vi "NI GetWaveform Queue.vi"(0 "Acq ID In":refnum<k15>, 1 "File Array":refnum<file>[](array[refnum]), 2 "timeout":dbl=1.0, 5 "Num Samps":i32=1000, 7 "Channel array":string[](array[string])=["0", "1"], 9 "Num Segs":i32=1, 11 "error in":errorcluster, 12 "Reverse?":bool, 13 "File Array":string[](array[string])) -> (4 "Acq ID Out":refnum<k15>, 15 "error out":errorcluster)   [LabVIEW 2022 SP3]
uses:
  <instrlib>/niScope/Acquire/Fetch/niScope Multi Fetch Binary 8.vi
  -ScanSystem/DataHandling/ReverseDataI8.vi
panel:
  # "Mujst convert data at output for Integers"
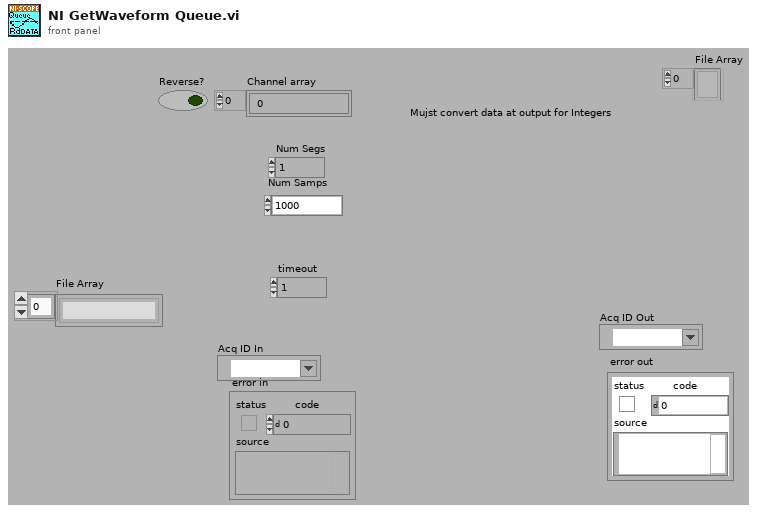
[diagram p1: front panel]
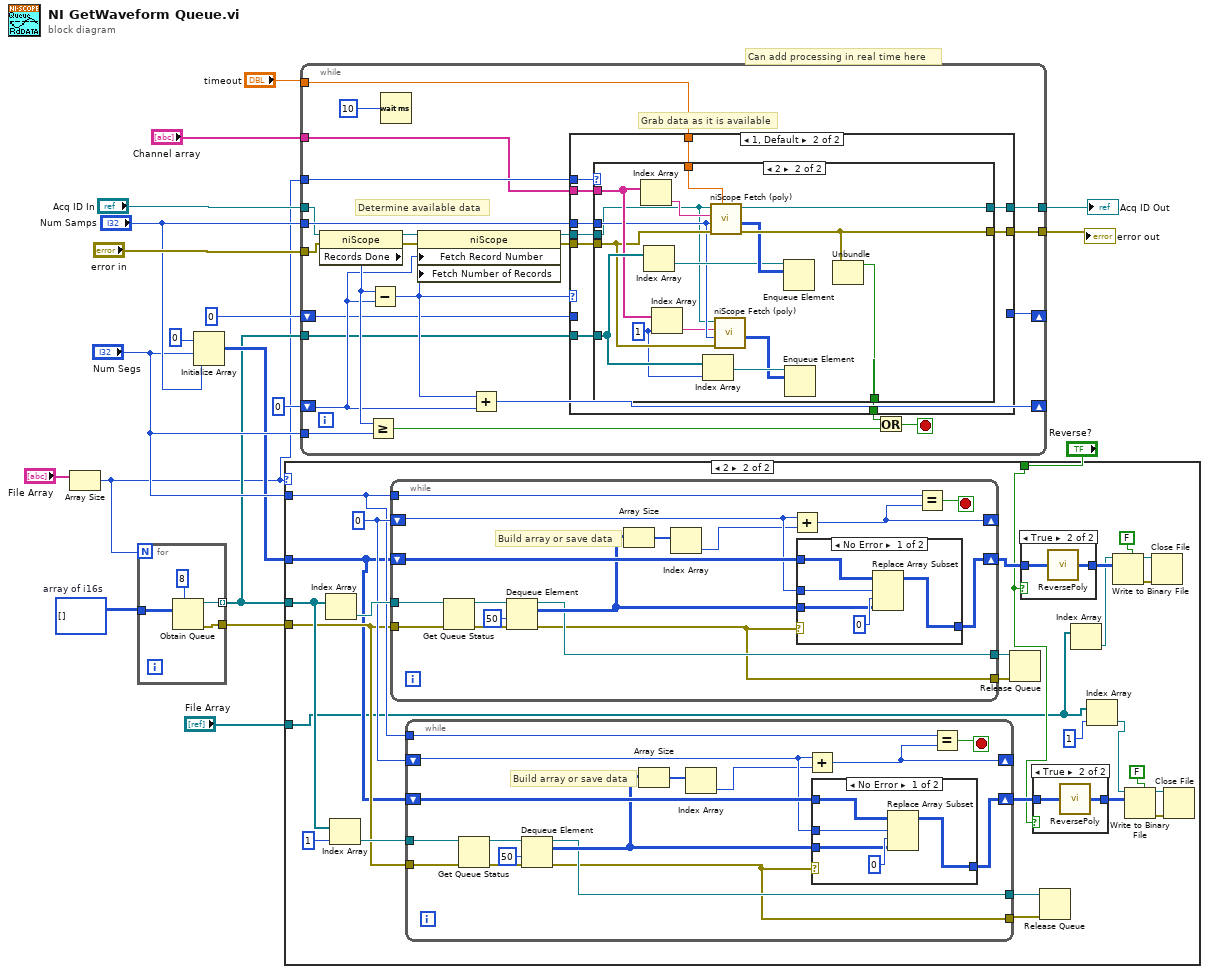
[diagram p0: block diagram]
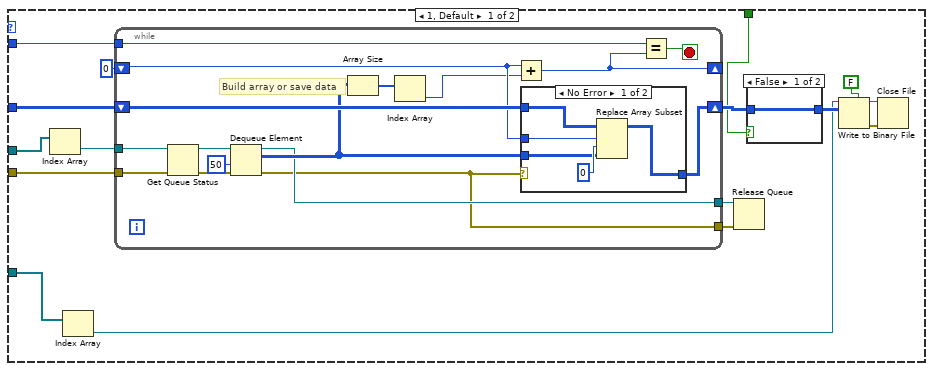
[diagram p2: hidden frame]
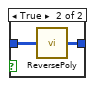
[diagram p3: hidden frame]
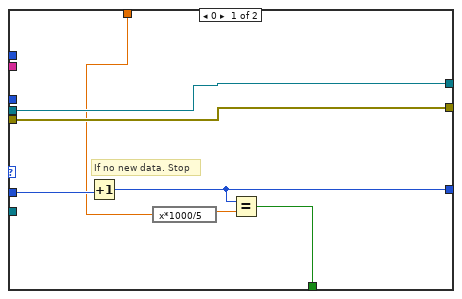
[diagram p9: hidden frame]
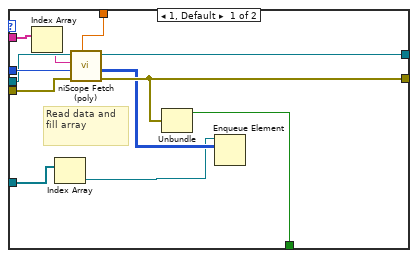
[diagram p10: hidden frame]
diagram:
  w11 = i8[][] []  # array of i16s
  # "Can add processing in real time here"
  n1 = Array Size(array="File Array") -> (size(s)=w1:i32)
  n2 = for {
    N: w1 -> [_]
    tunnel: w11 -> [w23]
    tunnel: [w21] -> w10
    tunnel: [w20] -> w8 mode=indexing
    n3 = Obtain Queue(max queue size (-1, unlimited)=8, element data type=w23) -> (queue out=w20:refnum<queue>, error out=w21:errorcluster)  [unwired: 2 in, 2 out]
  }
  n4 = Initialize Array(i8 0, "Num Segs", "Num Samps") -> (w9:i8[][])
  n5 = case shown="2" w1 {
    tunnel: "Num Segs" -> [w39 w82]
    tunnel: w10 -> [w38 w80]
    tunnel: w9 -> [w37 w70]
    tunnel: w8 -> [w33 w85]
    tunnel: "Reverse?" -> [w26 w69]
    tunnel: "File Array" -> [w25 w67]
    frame 1, Default {
      n6 = Index Array(array=w33) -> (element=w32:refnum<queue>)  [unwired: 1 in]
      n7 = Index Array(array=w25) -> (element=w24:refnum<file>)  [unwired: 1 in]
      n8 = while {
        tunnel: w32 -> [w58]
        tunnel: w38 -> [w57]
        shift-right: [w52] -> w27
        shift-left: w37 -> [w53]
        shift-right: [w46] -> _
        shift-left: 0 -> [w44]
        tunnel: [w49] -> w35
        tunnel: [w48] -> w34
        tunnel: w39 -> [w45]
        stop <- w47 stop-if-true
        # "Build array or save data"
        n9 = Get Queue Status(queue=w58, error in (no error)=w57) -> (queue out=w56:refnum<queue>, error out=w55:errorcluster)  [unwired: 7 out]
        n10 = Dequeue Element(queue=w56, timeout in ms (-1)=50, error in (no error)=w55) -> (queue out=w49:refnum<queue>, element=w51:i8[][], error out=w48:errorcluster)  [unwired: 1 out]
        n11 = Array Size(array=w51) -> (size(s)=w50:i32[])
        n12 = Index Array(array=w50) -> (element=w43:i32)  [unwired: 1 in]
        n13 = Add(x=w44, y=w43) -> (x+y=w46:i32)
        n14 = case shown="No Error" w48 {
          tunnel: w53 -> [w63 w64]
          tunnel: [w62 w64] -> w52
          tunnel: w51 -> [w59 _]
          tunnel: w44 -> [w61 _]
          frame No Error {
            n15 = Replace Array Subset(array=w63, new element=w59, index (row)=w61, index (col)=0) -> (w62:i8[][])
          }
          frame Error {
          }
        }
        n16 = Equal?(x=w45, y=w46) -> (x = y?=w47:bool)
      }
      n17 = Release Queue(queue=w35, error in (no error)=w34) -> ()  [unwired: 4 out]
      n18 = case shown="False" w26 {
        tunnel: [w40 w42] -> w28
        tunnel: w27 -> [w40 w41]
        frame False {
        }
        frame True {
          n19 = call-poly "ReversePoly.vi"("Array in"=w41) -> ("Array out"=w42:i8[][])
        }
      }
      n20 = Write to Binary File(file (use dialog)=w24, data=w28, 5:FALSE ("prepend array or string size? (T)")) -> (refnum out=w30:refnum<file>, error out=w29:errorcluster)  [unwired: 2 in, 2 out]
      n21 = Close File(refnum=w30, error in=w29) -> ()  [unwired: 2 out]
    }
    frame 2 {
      w83 = 0
      n22 = Index Array(array=w85) -> (element=w86:refnum<queue>)  [unwired: 1 in]
      n23 = Index Array(array=w85, index=1) -> (element=w81:refnum<queue>)
      n24 = while {
        tunnel: w86 -> [w135]
        tunnel: w80 -> [w134]
        shift-right: [w129] -> w77
        shift-left: w70 -> [w130]
        shift-right: [w123] -> _
        shift-left: w83 -> [w121]
        tunnel: [w126] -> w91
        tunnel: [w125] -> w90
        tunnel: w82 -> [w122]
        stop <- w124 stop-if-true
        # "Build array or save data"
        n25 = Get Queue Status(queue=w135, error in (no error)=w134) -> (queue out=w133:refnum<queue>, error out=w132:errorcluster)  [unwired: 7 out]
        n26 = Dequeue Element(queue=w133, timeout in ms (-1)=50, error in (no error)=w132) -> (queue out=w126:refnum<queue>, element=w128:i8[][], error out=w125:errorcluster)  [unwired: 1 out]
        n27 = Array Size(array=w128) -> (size(s)=w127:i32[])
        n28 = Index Array(array=w127) -> (element=w120:i32)  [unwired: 1 in]
        n29 = Add(x=w121, y=w120) -> (x+y=w123:i32)
        n30 = case shown="No Error" w125 {
          tunnel: w130 -> [w140 w141]
          tunnel: [w139 w141] -> w129
          tunnel: w128 -> [w136 _]
          tunnel: w121 -> [w138 _]
          frame No Error {
            n31 = Replace Array Subset(array=w140, new element=w136, index (row)=w138, index (col)=0) -> (w139:i8[][])
          }
          frame Error {
          }
        }
        n32 = Equal?(x=w122, y=w123) -> (x = y?=w124:bool)
      }
      n33 = while {
        tunnel: w81 -> [w113]
        tunnel: w80 -> [w112]
        shift-right: [w107] -> w71
        shift-left: w70 -> [w108]
        shift-right: [w101] -> _
        shift-left: w83 -> [w99]
        tunnel: [w104] -> w79
        tunnel: [w103] -> w78
        tunnel: w82 -> [w100]
        stop <- w102 stop-if-true
        # "Build array or save data"
        n34 = Get Queue Status(queue=w113, error in (no error)=w112) -> (queue out=w111:refnum<queue>, error out=w110:errorcluster)  [unwired: 7 out]
        n35 = Dequeue Element(queue=w111, timeout in ms (-1)=50, error in (no error)=w110) -> (queue out=w104:refnum<queue>, element=w106:i8[][], error out=w103:errorcluster)  [unwired: 1 out]
        n36 = Array Size(array=w106) -> (size(s)=w105:i32[])
        n37 = Index Array(array=w105) -> (element=w98:i32)  [unwired: 1 in]
        n38 = Add(x=w99, y=w98) -> (x+y=w101:i32)
        n39 = case shown="No Error" w103 {
          tunnel: w108 -> [w118 w119]
          tunnel: [w117 w119] -> w107
          tunnel: w106 -> [w114 _]
          tunnel: w99 -> [w116 _]
          frame No Error {
            n40 = Replace Array Subset(array=w118, new element=w114, index (row)=w116, index (col)=0) -> (w117:i8[][])
          }
          frame Error {
          }
        }
        n41 = Equal?(x=w100, y=w101) -> (x = y?=w102:bool)
      }
      n42 = Release Queue(queue=w91, error in (no error)=w90) -> ()  [unwired: 4 out]
      n43 = case shown="True" w69 {
        tunnel: [w95 w97] -> w76
        tunnel: w77 -> [w95 w96]
        frame False {
        }
        frame True {
          n44 = call-poly "ReversePoly.vi"("Array in"=w96) -> ("Array out"=w97:i8[][])
        }
      }
      n45 = case shown="True" w69 {
        tunnel: [w92 w94] -> w72
        tunnel: w71 -> [w92 w93]
        frame False {
        }
        frame True {
          n46 = call-poly "ReversePoly.vi"("Array in"=w93) -> ("Array out"=w94:i8[][])
        }
      }
      n47 = Release Queue(queue=w79, error in (no error)=w78) -> ()  [unwired: 4 out]
      n48 = Index Array(array=w67) -> (element=w68:refnum<file>)  [unwired: 1 in]
      n49 = Index Array(array=w67, index=1) -> (element=w66:refnum<file>)
      n50 = Write to Binary File(file (use dialog)=w68, data=w76, 5:FALSE ("prepend array or string size? (T)")) -> (refnum out=w88:refnum<file>, error out=w87:errorcluster)  [unwired: 2 in, 2 out]
      n51 = Write to Binary File(file (use dialog)=w66, data=w72, 5:FALSE ("prepend array or string size? (T)")) -> (refnum out=w74:refnum<file>, error out=w73:errorcluster)  [unwired: 2 in, 2 out]
      n52 = Close File(refnum=w88, error in=w87) -> ()  [unwired: 2 out]
      n53 = Close File(refnum=w74, error in=w73) -> ()  [unwired: 2 out]
    }
  }
  n54 = while {
    tunnel: [w165] -> w3
    tunnel: [w151] -> w2
    tunnel: "error in" -> [w155]
    tunnel: "Num Samps" -> [w164]
    tunnel: "Channel array" -> [w142]
    tunnel: "Acq ID In" -> [w162]
    tunnel: "timeout" -> [w163]
    shift-right: [w157] -> _
    shift-left: 0 -> [w148]
    tunnel: "Num Segs" -> [w158]
    shift-right: [w147] -> _
    shift-left: 0 -> [w146]
    tunnel: w8 -> [w144]
    tunnel: w1 -> [w143]
    stop <- w153 stop-if-true
    # "Grab data as it is available"
    # "Determine available data"
    n55 = property class="niScope"(reference=w162, error in=w155) -> (reference out=w160:refnum<k15>, error out=w161:errorcluster, "Records Done"=w154:i32)
    n56 = Greater Or Equal?(x=w154, y=w158) -> (x >= y?=w152:bool)
    n57 = Subtract(x=w154, y=w148) -> (x-y=w149:i32)
    n58 = Wait (ms)(milliseconds to wait=10) -> ()  [unwired: 1 out]
    n59 = property class="niScope"(reference=w160, error in=w161, "Fetch Record Number"=w148, "Fetch Number of Records"=w149) -> (reference out=w159:refnum<k15>, error out=w156:errorcluster)
    n60 = Add(x=w149, y=w148) -> (x+y=w157:i32)
    n61 = case shown="1, Default" w149 {
      tunnel: [w172 w182] -> w165
      tunnel: w164 -> [_ w181]
      tunnel: w163 -> [w167 w180]
      tunnel: w159 -> [w172 w175]
      tunnel: w156 -> [w171 w179]
      tunnel: [w171 w178] -> w151
      tunnel: [w168 w177] -> w150
      tunnel: [w166 _] -> w147
      tunnel: w146 -> [w170 _]
      tunnel: w144 -> [_ w176]
      tunnel: w143 -> [_ w174]
      tunnel: w142 -> [_ w173]
      frame 0 {
        # "If no new data. Stop"
        n62 = Increment(x=w170) -> (x+1=w166:i32)
        n63 = expression code="x*1000/5"(w167) -> (w169:dbl)
        n64 = Equal?(x=w166, y=w169) -> (x = y?=w168:bool)
      }
      frame 1, Default {
        n65 = case shown="2" w174 {
          tunnel: [w194 w210] -> w182
          tunnel: w181 -> [w193 w198]
          tunnel: w180 -> [w192 w209]
          tunnel: w179 -> [w191 w199]
          tunnel: [w190 w208] -> w178
          tunnel: [w189 w207] -> w177
          tunnel: w176 -> [w186 w201]
          tunnel: w175 -> [w188 w196]
          tunnel: w173 -> [w184 w200]
          frame 1, Default {
            # "Read data and fill array"
            n66 = Index Array(array=w184) -> (element=w183:string)  [unwired: 1 in]
            n67 = Index Array(array=w186) -> (element=w185:refnum<queue>)  [unwired: 1 in]
            n68 = call-poly <instrlib>:"niScope Fetch (poly).vi"("timeout"=w192, "error in"=w191, "numSamples"=w193, "channels"=w183, "instrument handle"=w188) -> ("error out"=w190:errorcluster, "wfm"=w187:i8[][], "instrument handle out"=w194:refnum<k15>)  [unwired: 4 out]
            n69 = Unbundle(w190) -> ("status"=w189:bool)  [unwired: 2 out]
            n70 = Enqueue Element(queue=w185, element=w187) -> ()  [unwired: 1 in, 4 out]
          }
          frame 2 {
            w195 = 1
            n71 = Index Array(array=w200) -> (element=w204:string)  [unwired: 1 in]
            n72 = Index Array(array=w201) -> (element=w205:refnum<queue>)  [unwired: 1 in]
            n73 = Index Array(array=w200, index=w195) -> (element=w197:string)
            n74 = Index Array(array=w201, index=w195) -> (element=w203:refnum<queue>)
            n75 = call-poly <instrlib>:"niScope Fetch (poly).vi"("timeout"=w209, "error in"=w199, "numSamples"=w198, "channels"=w204, "instrument handle"=w196) -> ("error out"=w208:errorcluster, "wfm"=w206:i8[][], "instrument handle out"=w210:refnum<k15>)  [unwired: 4 out]
            n76 = call-poly <instrlib>:"niScope Fetch (poly).vi"("error in"=w199, "numSamples"=w198, "channels"=w197, "instrument handle"=w196) -> ("wfm"=w202:i8[][])  [unwired: 1 in, 6 out]
            n77 = Enqueue Element(queue=w205, element=w206) -> ()  [unwired: 1 in, 4 out]
            n78 = Enqueue Element(queue=w203, element=w202) -> ()  [unwired: 1 in, 4 out]
            n79 = Unbundle(w208) -> ("status"=w207:bool)  [unwired: 2 out]
          }
        }
      }
    }
    n80 = Or(x=w150, y=w152) -> (x .or. y?=w153:bool)
  }
  "error out" <- w2
  "Acq ID Out" <- w3
